vi "XY Graph Shift Multiple Plots.vi"(6 "Plot Shift Parameters":T1 caption="IRF Analysis Parameters", 7 "Reference Decay":cluster{"t Array":dbl[], "I Array":dbl[]}, 8 "error in (no error)":errorcluster, 10 "Selected Plots":i32[](array[numeric]), 11 "Selected Plot Info":T3) -> (0 "error out":errorcluster, 1 "Shifted Plot Message":string, 3 "Last Shifted Plot":cluster{"t Array":dbl[], "IRF Array":dbl[]}, 4 "Single Plot?":bool)   [LabVIEW 2021, in "XY Graph Add-Ons.lvlib"]
uses:
  XY Graph Add-Ons.lvlib
  XY Graph Selected Plot Info.ctl
  XY Graph Refnum.ctl
  <vilib>/Utility/miscctls.llb/LVPoint32TypeDef.ctl
  XY Graph Plot Shift Parameters.ctl
  XY Graph Plot Shift Method.ctl
  Strings/Strings.lvlib
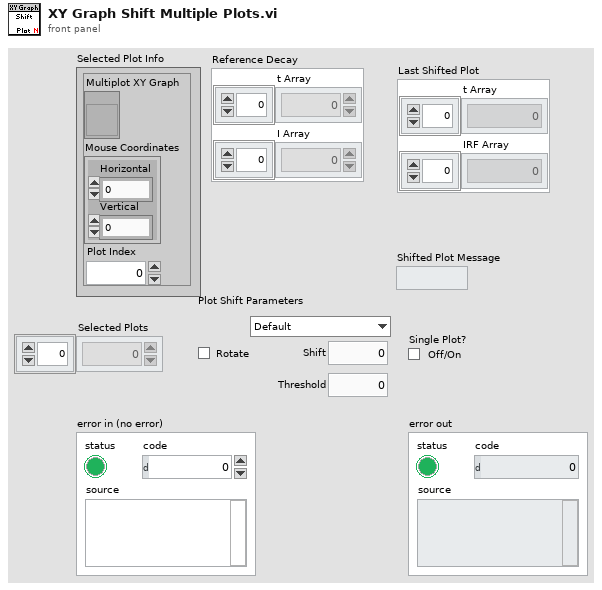
[diagram p1: front panel]
types:
  T1 = typedef "XY Graph Add-Ons.lvlib/XY Graph Plot Shift Parameters.ctl" = cluster{"Type":T2, "Shift":dbl[unit], "Threshold":dbl, "Rotate":bool}
  T2 = typedef "XY Graph Add-Ons.lvlib/XY Graph Plot Shift Method.ctl" = enum16{"Default", "CFD", "Threshold", "Cross-Correlation"}
  T3 = typedef "XY Graph Add-Ons.lvlib/XY Graph Selected Plot Info.ctl" = cluster{"Multiplot XY Graph":T4, "Mouse Coordinates":T5, "Plot Index":i32}
  T4 = typedef "XY Graph Add-Ons.lvlib/XY Graph Refnum.ctl" = refnum<vi>
  T5 = typedef "LVPoint32TypeDef.ctl" = cluster{"Horizontal":i32, "Vertical":i32}
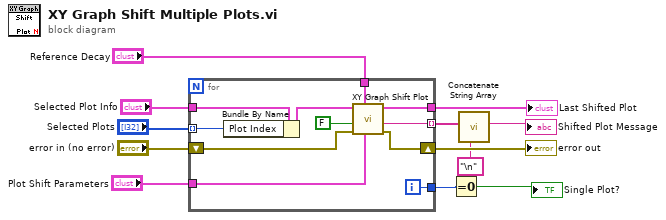
[diagram p0: block diagram]
diagram:
  n1 = for {
    tunnel: "Selected Plot Info" -> [w23]
    tunnel: [w21] -> w7 mode=indexing
    tunnel: [w19] -> w9
    shift-right: [w20] -> w10
    shift-left: "error in (no error)" -> [w22]
    tunnel: "Selected Plots" -> [w17] mode=indexing
    tunnel: [w16] -> w4
    tunnel: "Reference Decay" -> [w14]
    tunnel: "Plot Shift Parameters" -> [w13]
    i -> [w16]
    n2 = Bundle By Name(cluster=w23, "Plot Index"=w17) -> (w18:T3)
    n3 = call "XY Graph Shift Plot.vi"("Plot Shift Parameters"=w13, "Reference Decay"=w14, "error in (no error)"=w22, "Replace Plot (T)?"=FALSE, "Selected Plot Info"=w18) -> ("Error Out"=w20:errorcluster, "Shift Decay Message"=w21:string, "Shifted Plot"=w19:cluster{"t Array":dbl[], "IRF Array":dbl[]})  [unwired: 4 in]
  }
  "error out" <- w10
  "Last Shifted Plot" <- w9
  n4 = Equal To 0?(x=w4) -> (x = 0?=→"Single Plot?":bool)
  n5 = call "Concatenate String Array.vi"("Separator (TAB)"="\n", "String Array"=w7) -> ("Formatted String"=→"Shifted Plot Message":string)  [unwired: 9 in]
